vi "Update From Result.vi"(8 "error in (no error)":errorcluster, 10 "Result Row":refnum<class "Result Row.lvclass">, 11 "Game in":refnum<class "Game.lvclass">) -> (0 "error out":errorcluster, 3 "Game out":refnum<class "Game.lvclass">)   [LabVIEW 2022 SP3]
uses:
  Game.lvclass
  Conditum/Result Row/Result Row.lvclass
  Game.lvclass/Game.ctl
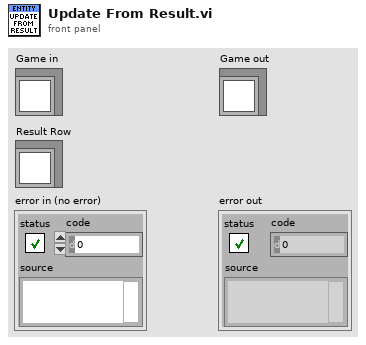
[diagram p1: front panel]
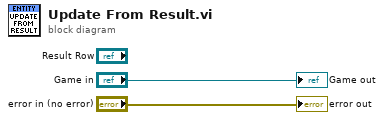
[diagram p0: block diagram]
diagram:
  "error out" <- "error in (no error)"
  "Game out" <- "Game in"
